vi "GetParameterDefaults.vi"(8 "error in (no error)":errorcluster, 11 "CDefaultRuleFileParser in":refnum<class "CDefaultRuleFileParser.lvclass">) -> (0 "error out":errorcluster, 1 "Parameter defaults":string, 3 "CDefaultRuleFileParser out":refnum<class "CDefaultRuleFileParser.lvclass">)   [LabVIEW 2020, in "DefaultExtensions.lvlib" / "CDefaultRuleFileParser.lvclass"]
uses:
  CDefaultRuleFileParser.lvclass
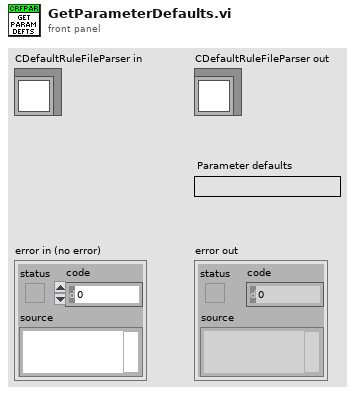
[diagram p1: front panel]
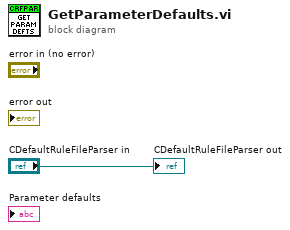
[diagram p0: block diagram]
diagram:
  "CDefaultRuleFileParser out" <- "CDefaultRuleFileParser in"
